vi "file status Write.vi"(4 "error in (no error)":errorcluster, 5 "Value":bool[][](array[boolean]), 6 "Container State":T6, 7 "Display State In":T1={"Nspeakers"=13, "actions"=[], "Wspeaker"=13, "Wmic"=13, "sel mic"=13, "hover"={"type"=enum."None", "index"=0}, "locked"=FALSE, "states"=[], "sel speak"=13, "selected"=refnum, "Events"={"Mic change"=refnum, "Selection change"=refnum}}) -> (0 "error out":errorcluster, 3 "Display State Out":T1={"Nspeakers"=13, "actions"=[], "Wspeaker"=13, "Wmic"=13, "sel mic"=13, "hover"={"type"=enum."None", "index"=0}, "locked"=FALSE, "states"=[], "sel speak"=13, "selected"=refnum, "Events"={"Mic change"=refnum, "Selection change"=refnum}})   [LabVIEW 2015, in "HRTF Config.xctl"]
uses:
  HRTF Config.xctl
  <vilib>/_xctls/Container State.ctl
  State.vi
  Hover Data.ctl
  Hover Item.ctl
  Speaker State.ctl
  Events.ctl
  Selection changed.ctl
  <vilib>/_xctls/XControlSupport.lvlib
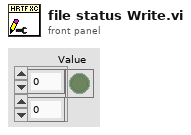
[diagram p1: front panel]
types:
  T1 = typedef "HRTF Config.xctl/State.vi" = cluster{"Nspeakers":i32, "actions":string[], "Wspeaker":i32, "Wmic":i32, "sel mic":i32, "hover":T2, "locked":bool, "states":T4[], "sel speak":i32, "selected":refnum<vi>, "Events":T5}
  T2 = typedef "HRTF Config.xctl/Hover Data.ctl" = cluster{"type":T3, "index":i32}
  T3 = typedef "HRTF Config.xctl/Hover Item.ctl" = enum16{"None", "Speaker", "Mic"}
  T4 = typedef "HRTF Config.xctl/Speaker State.ctl" = cluster{"right cal":bool, "left cal":bool, "selected":bool}
  T5 = typedef "HRTF Config.xctl/Events.ctl" = cluster{"Mic change":refnum<user-event>, "Selection change":refnum<user-event>}
  T6 = typedef "XControlSupport.lvlib/Container State.ctl" = cluster{"Indicator?":bool, "Run Mode?":bool, " Refnum":refnum<vi>}
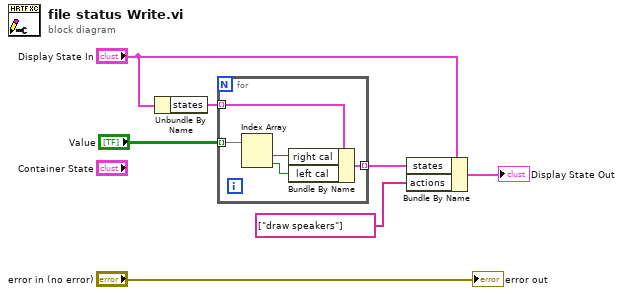
[diagram p0: block diagram]
diagram:
  n1 = Unbundle By Name("Display State In") -> ("states"=w4:T4[])
  n2 = for {
    tunnel: w4 -> [w11] mode=indexing
    tunnel: "Value" -> [w12] mode=indexing
    tunnel: [w8] -> w2 mode=indexing
    n3 = Index Array(array=w12) -> (element #1=w10:bool, element #2=w9:bool)  [unwired: 2 in]
    n4 = Bundle By Name(cluster=w11, "right cal"=w10, "left cal"=w9) -> (w8:T4)
  }
  n5 = Bundle By Name(cluster="Display State In", "states"=w2, "actions"=string[] ["draw speakers"]) -> (→"Display State Out":T1)
  "error out" <- "error in (no error)"
